vi "check_mux_is_connected.vi"(3 "error in (no error)":errorcluster) -> (1 "error?":bool)   [LabVIEW 2016]
uses:
  <vilib>/Utility/error.llb/DialogType.ctl
  <instrlib>/QuickMux/QuickMux.lvlib
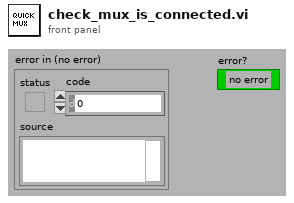
[diagram p1: front panel]
types:
  T1 = typedef "DialogType.ctl" = u16
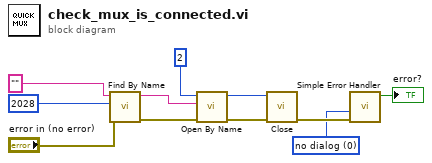
[diagram p0: block diagram]
diagram:
  w1 = T1 0 items=["no dialog", "OK message", "continue or stop message", "OK message + warnings", "continue/stop + warnings"] ("type of dialog (OK msg:1)")
  n1 = call <instrlib>:"Find By Name.vi"("error in (no error)"="error in (no error)", "length"=u16 2028, "nameList"="") -> ("error out"=w8:errorcluster, "nameList out"=w9:string)  [unwired: 5 in, 2 out]
  n2 = call <instrlib>:"Open By Name.vi"("error in (no error)"=w8, "deviceName"=w9, "handle 2"=u64 2) -> ("error out"=w4:errorcluster, "handle"=w5:u64)  [unwired: 6 in, 1 out]
  n3 = call <instrlib>:"Close.vi"("error in (no error)"=w4, "handle"=w5) -> ("error out"=w2:errorcluster)  [unwired: 8 in, 1 out]
  n4 = call <vilib>:"Simple Error Handler.vi"("type of dialog (OK msg:1)"=w1, "error in (no error)"=w2) -> ("error?"=→"error?":bool)  [unwired: 3 in, 4 out]
